vi "errorMasage.vi"(1 "error (h)":bool, 2 "millisecond timer value":u32, 3 "Boolean":bool, 4 "error message":refnum<vi>) -> (0 "millisecond timer value 2":u32)   [LabVIEW 2013]
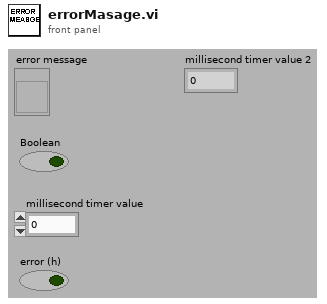
[diagram p1: front panel]
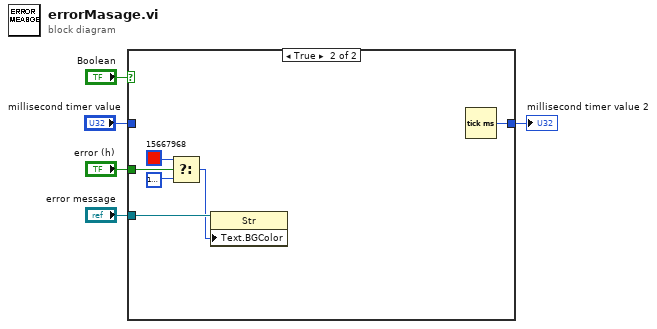
[diagram p0: block diagram]
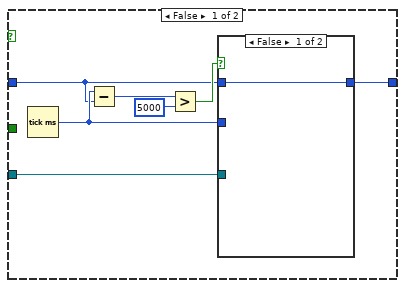
[diagram p2: hidden frame]
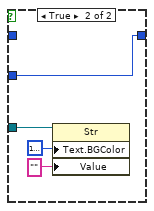
[diagram p3: hidden frame]
diagram:
  n1 = case shown="True" "Boolean" {
    tunnel: [w7 w23] -> w1
    tunnel: "millisecond timer value" -> [w6 _]
    tunnel: "error message" -> [w9 w22]
    tunnel: "error (h)" -> [_ w18]
    frame False {
      n2 = Tick Count (ms)() -> (millisecond timer value=w8:u32)
      n3 = Subtract(x=w8, y=w6) -> (x-y=w12:u32)
      n4 = Greater?(x=w12, y=u32 5000) -> (0:w10:bool)
      n5 = case shown="False" w10 {
        tunnel: w9 -> [_ w17]
        tunnel: w8 -> [_ w14]
        tunnel: [w13 w14] -> w7
        tunnel: w6 -> [w13 _]
        frame False {
        }
        frame True {
          n6 = property class="Str"(reference=w17, "Text.BGColor"=u32 16777238, "Value"="") -> ()  [unwired: 1 in, 2 out]
        }
      }
    }
    frame True {
      n7 = Select(t=u32 15667968, s=w18, f=u32 16777238) -> (s? t:f=w19:u32)
      n8 = property class="Str"(reference=w22, "Text.BGColor"=w19) -> ()  [unwired: 1 in, 2 out]
      n9 = Tick Count (ms)() -> (millisecond timer value=w23:u32)
    }
  }
  "millisecond timer value 2" <- w1
